vi "init.vi"(8 "error in (no error)":errorcluster, 11 "WindowsTarget in":refnum<class "WindowsTarget.lvclass">) -> (0 "error out":errorcluster, 3 "WindowsTarget out":refnum<class "WindowsTarget.lvclass">)   [LabVIEW 2012, in "WindowsTarget.lvclass"]
doc: "Initializes object."
uses:
  WindowsTarget.lvclass
  WindowsTarget.lvclass/WindowsTarget.ctl
  C/Program Files (x86)/National Instruments/LabVIEW 2012/user.lib/Common/ComponentModel/ComponentModelRT/LoopTimer/ILoopTimer/ILoopTimer.lvclass
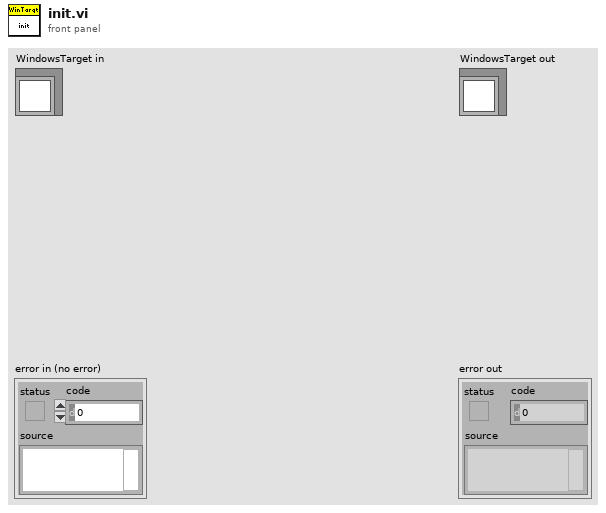
[diagram p1: front panel]
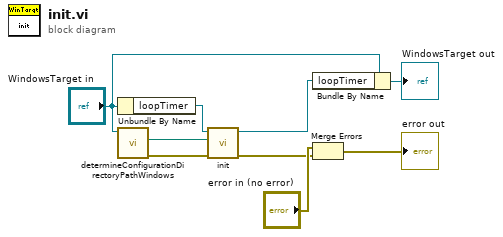
[diagram p0: block diagram]
diagram:
  n1 = Unbundle By Name("WindowsTarget in") -> ("loopTimer"=w8:refnum<class "ILoopTimer.lvclass">)
  n2 = call-dynamic "determineConfigurationDirectoryPathWindows.vi"("WindowsTarget in"="WindowsTarget in") -> ("error out"=w1:errorcluster, "configDirectoryPathWindows"=w3:path)  [unwired: 8 in, 1 out]
  n3 = call-dynamic "init.vi"("error in (no error)"=w1, "configDirectoryPathWindows"=w3, "ILoopTimer in"=w8) -> ("error out"=w5:errorcluster, "ILoopTimer out"=w7:refnum<class "ILoopTimer.lvclass">)  [unwired: 7 in]
  n4 = Bundle By Name(cluster="WindowsTarget in", "loopTimer"=w7) -> (→"WindowsTarget out":refnum<class "WindowsTarget.lvclass">)
  n5 = Merge Errors("error in (no error)", w5) -> (→"error out":errorcluster)
